vi "svx_Polar_Manage_Cluster.vi"(10 "index":i32, 11 "Clust Refnum":refnum<vi>) -> ()   [LabVIEW 2017, in "SVX Polar Plot.xctl"]
uses:
  <vilib>/addons/_XControls/Polar Plot/SVX Polar Plot.xctl
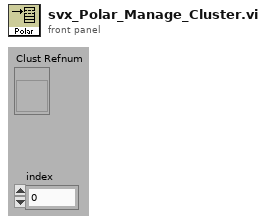
[diagram p1: front panel]
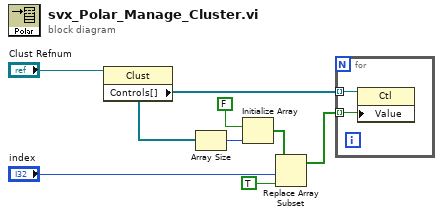
[diagram p0: block diagram]
diagram:
  n1 = property on="Property Node" class="Clust"(reference="Clust Refnum") -> ("Controls[]"=w3:refnum<vi>[])  [unwired: 1 in, 2 out]
  n2 = Array Size(array=w3) -> (size(s)=w6:i32)
  n3 = Initialize Array(FALSE ("Caption visible"), w6) -> (w4:bool[])
  n4 = Replace Array Subset(array=w4, new element=TRUE ("new element/subarray"), index="index") -> (w2:bool[])
  n5 = for {
    tunnel: w2 -> [w9] mode=indexing
    tunnel: w3 -> [w10] mode=indexing
    n6 = property class="Ctl"(reference=w10, "Value"=w9) -> ()  [unwired: 1 in, 2 out]
  }
